vi "MRC Systemcore Get Battery Voltage.vi"(8 "error in (no error)":errorcluster) -> (0 "error out":errorcluster, 3 "voltage out":sgl)   [LabVIEW 2026, in "MrcLib.lvlib"]
doc: "MRC_Status MRC_CALLCONV MRC_Systemcore_GetBatteryVoltage(float* voltage);"
uses:
  MrcLib.lvlib
  MrcLib.dll
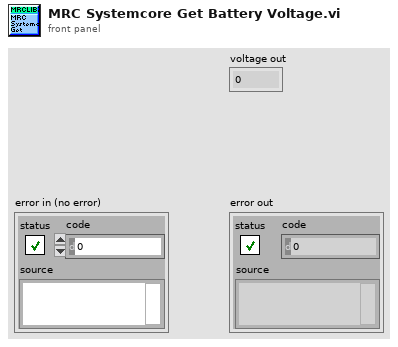
[diagram p1: front panel]
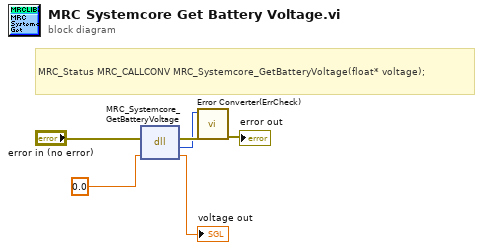
[diagram p0: block diagram]
diagram:
  # "MRC_Status MRC_CALLCONV MRC_Systemcore_GetBatteryVoltage(float* voltage);"
  n1 = dll-call lib="MrcLib.*" fn="MRC_Systemcore_GetBatteryVoltage"(error in="error in (no error)", "voltage"=sgl 0.0) -> (error out=w3:errorcluster, w1:i32, "voltage"=→"voltage out":sgl)  [unwired: 2 in, 1 out]
  n2 = call "Error Converter(ErrCheck).vi"("error in (no error)"=w3, "status"=w1) -> ("error out"=→"error out":errorcluster)  [unwired: 9 in]
